vi "Tab_003_PH.vi"() -> ()   [LabVIEW 2021]
panel:
  out "initialized array":dbl[](array[numeric])
  in  "dimension size":i32=5
  in  "element":dbl=3.0
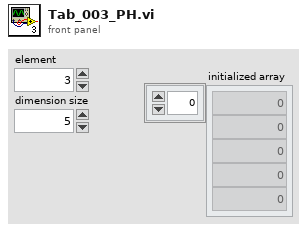
[diagram p1: front panel]
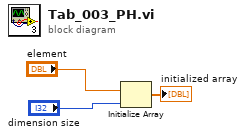
[diagram p0: block diagram]
diagram:
  n1 = Initialize Array("element", "dimension size") -> (→"initialized array":dbl[])
